vi "Create Resources.vi"(0 "instance":i16) -> (4 "channel collection builder":refnum<class "Collection Builder.lvclass">, 15 "niVST Common Reference FPGA.lvclass":refnum<class "niUSRP Rx Core v1 FPGA.lvclass">)   [LabVIEW 2025, in "niUSRP Rx Core v1 FPGA.lvclass"]
uses:
  niUSRP Rx Core v1 FPGA.lvclass
  <instrlib>/_niInstr/Instruction Framework/v1/FPGA/Collection Builder/Collection Builder.lvclass
  C:/Program Files/NI/LVAddons/niidl/1/instr.lib/_niInstr/Instruction Framework/v1/FPGA/Interfaces/Address Space/Address Space.lvclass
  niUSRP Rx Core v1 FPGA.lvclass/niUSRP Rx Core v1 FPGA.ctl
  <instrlib>/_niInstr/Instruction Framework/v1/FPGA/Helper Classes/Single Address Space Collection/Single Address Space Collection.lvclass
  C:/Program Files/NI/LVAddons/niidl/1/instr.lib/_niInstr/Instruction Framework/v1/FPGA/Interfaces/Address Space Collection/Address Space Collection.lvclass
  <vilib>/rvi/DataTransferAndStorage/Container/Common/niFpgaContainerGetUniqueNameForEmu.vi
  <vilib>/rvi/DataTransferAndStorage/Container/Common/niFpgaContainerSetEmuInfo.vi
  <vilib>/rvi/eio/common/nirviEmuReportErrorAndStop.vi
  <vilib>/rvi/LocalResourceManager/LocalResourceManager.xnode
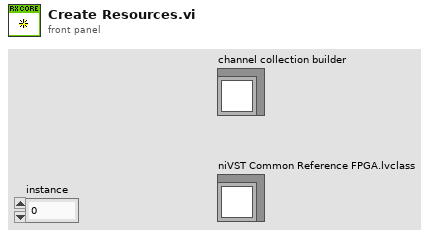
[diagram p1: front panel]
types:
  T1 = typedef "niInstr Address Space Collection Builder v1 FPGA.lvlib/Parent Metadata.ctl" = cluster{"UID":u16, "version":u16, "oldest compatible version":u16}
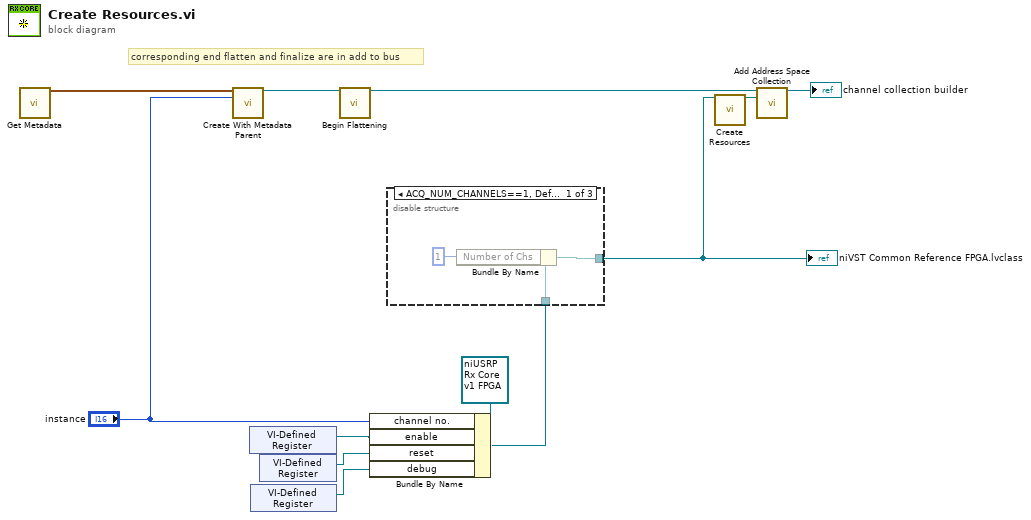
[diagram p0: block diagram]
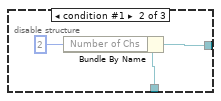
[diagram p2: hidden frame]
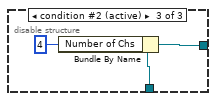
[diagram p3: hidden frame]
diagram:
  # "corresponding end flatten and finalize are in add to bus"
  n1 = call "Get Metadata.vi"() -> ("shared metadata"=w11:T1)  [unwired: 15 in]
  n2 = call <instrlib>:"Create With Metadata Parent.vi"("parent metadata"=w11, "instance (0)"="instance") -> ("collection builder"=w9:refnum<class "Collection Builder.lvclass">)  [unwired: 13 in]
  n3 = xnode "VI-Defined Register"() -> ("Register Out"=w7:refnum<k21>)
  n4 = xnode "VI-Defined Register"() -> ("Register Out"=w1:refnum<k21>)
  n5 = xnode "VI-Defined Register"() -> ("Register Out"=w6:refnum<k21>)
  n6 = call <instrlib>:"Begin Flattening.vi"("collection builder in"=w9) -> ("collection builder out"=w8:refnum<class "Collection Builder.lvclass">)  [unwired: 14 in]
  n7 = Bundle By Name(cluster=refnum<class "niUSRP Rx Core v1 FPGA.lvclass"> refnum ("niVST Common Reference FPGA.lvclass"), "channel no."="instance", "enable"=w7, "reset"=w6, "debug"=w1) -> (w4:refnum<class "niUSRP Rx Core v1 FPGA.lvclass">)
  n8 = disable-structure shown="ACQ_NUM_CHANNELS==1, Default" {
    disable-tunnel: [w15 w18 w21] -> w3
    disable-tunnel: w4 -> [w14 w17 w20]
    frame condition #0 {
      n9 = Bundle By Name(cluster=w14, "Number of Chs"=u8 1 ("rx regs.Number of Chs")) -> (w15:refnum<class "niUSRP Rx Core v1 FPGA.lvclass">)
    }
    frame condition #1 {
      n10 = Bundle By Name(cluster=w17, "Number of Chs"=u8 2 ("rx regs.Number of Chs")) -> (w18:refnum<class "niUSRP Rx Core v1 FPGA.lvclass">)
    }
    frame condition #2 (active) {
      n11 = Bundle By Name(cluster=w20, "Number of Chs"=u8 4 ("rx regs.Number of Chs")) -> (w21:refnum<class "niUSRP Rx Core v1 FPGA.lvclass">)
    }
  }
  "niVST Common Reference FPGA.lvclass" <- w3
  n12 = call <instrlib>:"Create Resources.vi"("address space"=w3) -> ("single address space collection"=w5:refnum<class "Single Address Space Collection.lvclass">)  [unwired: 14 in]
  n13 = call <instrlib>:"Add Address Space Collection.vi"("collection builder in"=w8, "address space collection"=w5) -> ("collection builder out"=→"channel collection builder":refnum<class "Collection Builder.lvclass">)  [unwired: 13 in]
